vi "CommonVIs_SetError.vi"(1 "status":bool, 2 "code (5000)":i32=5000, 3 "source":string, 5 "error in (no error)":errorcluster, 6 "UserDefinedCodes(+5000)":i32=-1) -> (19 "error out":errorcluster)   [LabVIEW 2020]
doc: "You can use this VI to generate errors."
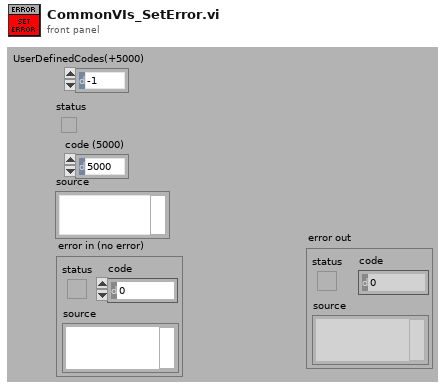
[diagram p1: front panel]
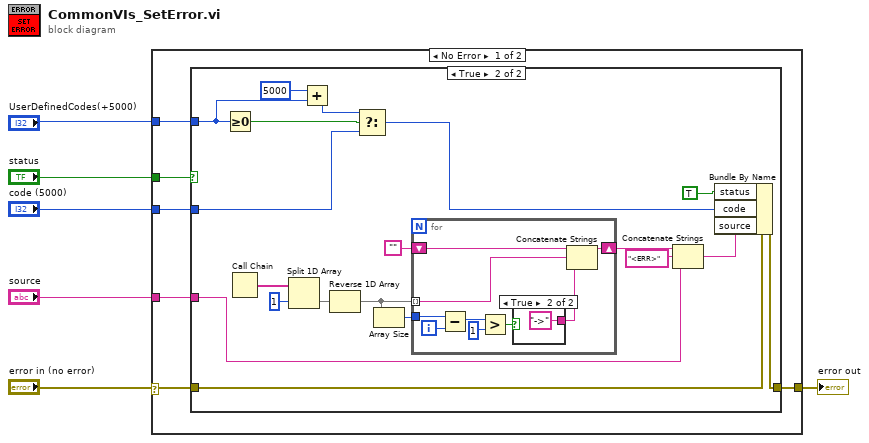
[diagram p0: block diagram]
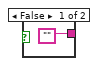
[diagram p3: hidden frame]
diagram:
  n1 = case shown="No Error" "error in (no error)" {
    selector: "error in (no error)" -> [w8 w44]
    tunnel: [w12 w44] -> w6
    tunnel: "status" -> [w11 _]
    tunnel: "code (5000)" -> [w10 _]
    tunnel: "source" -> [w9 _]
    tunnel: "UserDefinedCodes(+5000)" -> [w7 _]
    frame No Error {
      n2 = case shown="True" w11 {
        tunnel: w8 -> [w13 w32]
        tunnel: [w13 w31] -> w12
        tunnel: w10 -> [_ w18]
        tunnel: w9 -> [_ w22]
        tunnel: w7 -> [_ w16]
        frame False {
        }
        frame True {
          n3 = Greater Or Equal To 0?(x=w16) -> (x >= 0?=w19:bool)
          n4 = Call Chain() -> (call chain=w29:string[])
          n5 = Split 1D Array(array=w29, index=1) -> (second subarray=w27:string[])  [unwired: 1 out]
          n6 = Add(x=5000, y=w16) -> (x+y=w15:i32)
          n7 = Reverse 1D Array(array=w27) -> (reversed array=w20:string[])
          n8 = Select(t=w15, s=w19, f=w18) -> (s? t:f=w17:i32)
          n9 = Array Size(array=w20) -> (size(s)=w26:i32)
          n10 = for {
            shift-right: [w33] -> w24
            shift-left: "" -> [w36]
            tunnel: w20 -> [w34] mode=indexing
            tunnel: w26 -> [w41]
            i -> [w40]
            n11 = Subtract(x=w41, y=w40) -> (x-y=w39:i32)
            n12 = Greater?(x=w39, y=1) -> (0:w37:bool)
            n13 = case shown="True" w37 {
              tunnel: ["" "->"] -> w35
              frame False {
              }
              frame True {
              }
            }
            n14 = Concatenate Strings(w36, w34, w35) -> (w33:string)
          }
          n15 = Concatenate Strings(w24, "<ERR>" ("Substring"), w22) -> (w25:string)
          n16 = Bundle By Name(cluster=w32, "status"=TRUE ("Bundle Element"), "code"=w17, "source"=w25) -> (w31:errorcluster)
        }
      }
    }
    frame Error {
    }
  }
  "error out" <- w6
